vi "Rx Inline Start.vi"(8 "error in (no error)":errorcluster, 10 "Dispatcher Interface in":refnum<class "Dispatcher Interface.lvclass">, 11 "Plugin in":refnum<class "Plugin.lvclass">) -> (0 "error out":errorcluster, 2 "Dispatcher Interface out":refnum<class "Dispatcher Interface.lvclass">, 3 "Plugin out":refnum<class "Plugin.lvclass">)   [LabVIEW 2017, in "DSF Core.lvlib" / "Plugin.lvclass"]
uses:
  Plugin.lvclass
  Interface/Dispatcher/Dispatcher Interface.lvclass
  Plugin.lvclass/Plugin.ctl
  Interface/Dispatcher/Command.ctl
  Transfer Group/Transfer Group.lvclass
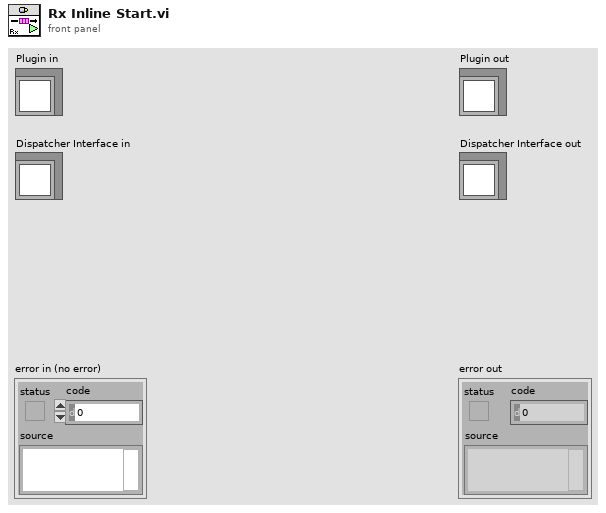
[diagram p1: front panel]
types:
  T1 = typedef "DSF Core.lvlib/Dispatcher Interface.lvclass/Command.ctl" = enum8{"Idle", "Start", "Rx", "Tx", "Set Inline Buffer", "Shutdown", "Error"}
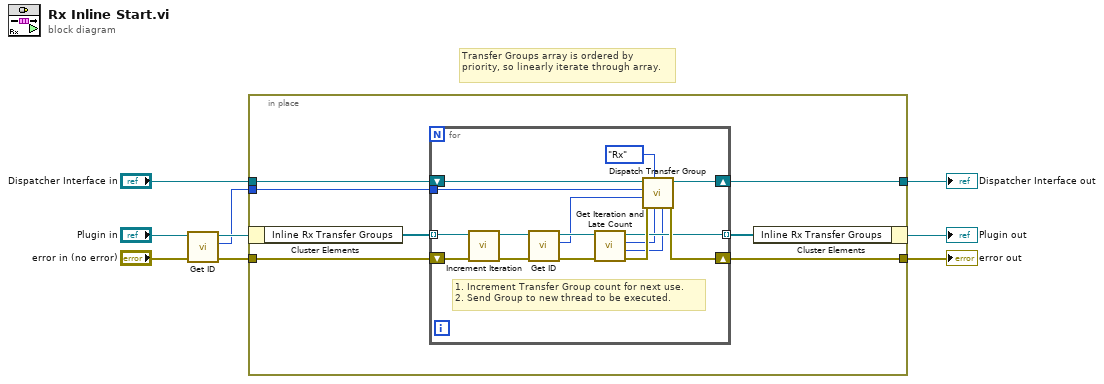
[diagram p0: block diagram]
diagram:
  # "Transfer Groups array is ordered by priority, so linearly iterate through array."
  n1 = call "Get ID.vi"("Plugin in"="Plugin in") -> ("id"=w2:i32, "Plugin out"=w3:refnum<class "Plugin.lvclass">)  [unwired: 9 in]
  n2 = in-place {
    in-place-border: "error in (no error)" -> [w15]
    in-place-border: [w14] -> w8
    in-place-border: "Dispatcher Interface in" -> [w11]
    in-place-border: w2 -> [w10]
    in-place-border: [w9] -> w1
    n3 = in-place-cluster #1(w3) -> ("Inline Rx Transfer Groups"=w13:refnum<class "Transfer Group.lvclass">[])
    n4 = for {
      tunnel: w13 -> [w26] mode=indexing
      shift-right: [w29] -> w14
      shift-left: w15 -> [w27]
      tunnel: [w21] -> w12 mode=indexing
      shift-right: [w24] -> w9
      shift-left: w11 -> [w25]
      tunnel: w10 -> [w23]
      # "1. Increment Transfer Group count for next use.\n2. Send Group to new thread to be executed."
      n5 = call "Increment Iteration.vi"("error in (no error)"=w27, "Transfer Group in"=w26) -> ("error out"=w28:errorcluster, "Transfer Group out"=w17:refnum<class "Transfer Group.lvclass">)  [unwired: 8 in]
      n6 = call "Get ID.vi"("Transfer Group in"=w17) -> ("id"=w20:i32, "Transfer Group out"=w22:refnum<class "Transfer Group.lvclass">)  [unwired: 9 in]
      n7 = call "Get Iteration and Late Count.vi"("error in (no error)"=w28, "Transfer Group in"=w22) -> ("error out"=w30:errorcluster, "late count"=w16:i32, "iteration"=w18:u64, "Transfer Group out"=w21:refnum<class "Transfer Group.lvclass">)  [unwired: 6 in]
      n8 = call "Dispatch Transfer Group.vi"("Late Count"=w16, "Iteration"=w18, "command"=Command."Rx", "error in (no error)"=w30, "Transfer Group ID"=w20, "Plugin ID"=w23, "Dispatcher Interface in"=w25) -> ("error out"=w29:errorcluster, "Dispatcher Interface out"=w24:refnum<class "Dispatcher Interface.lvclass">)  [unwired: 3 in]
    }
    n9 = in-place-cluster #1("Inline Rx Transfer Groups"=w12) -> (→"Plugin out":refnum<class "Plugin.lvclass">)
  }
  "error out" <- w8
  "Dispatcher Interface out" <- w1
